vi "requestStop.vi"(8 "error in (no error)":errorcluster, 11 "BoolUserEventStopMechanism In":refnum<class "BoolUserEventStopMechanism.lvclass">) -> (0 "error out":errorcluster, 3 "BoolUserEventStopMechanism Out":refnum<class "BoolUserEventStopMechanism.lvclass">)   [LabVIEW 2023, in "TLC_Daemon.lvlib" / "BoolUserEventStopMechanism.lvclass"]
doc: "Triggers a stop request for a target task.\n_____________________________________\nTLC Daemon 1.0.0.2\nCopyright (c) 2026 Andrea Cadei"
uses:
  BoolUserEventStopMechanism.lvclass
  BoolUserEventStopMechanism.lvclass/BoolUserEventStopMechanism.ctl
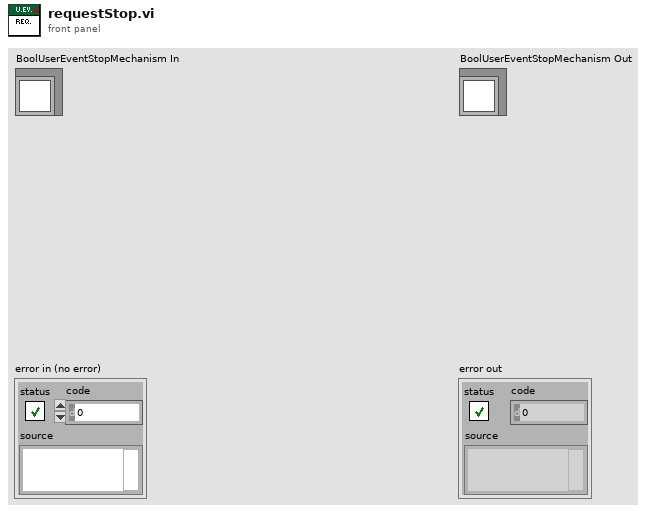
[diagram p1: front panel]
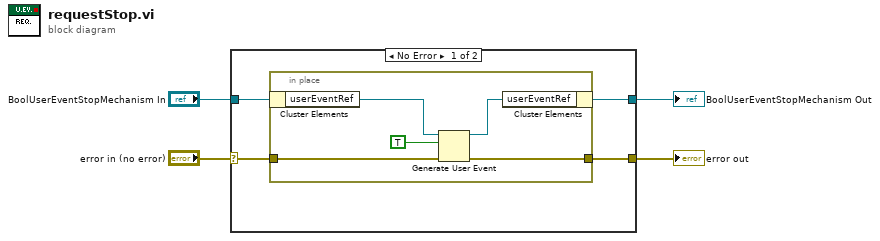
[diagram p0: block diagram]
diagram:
  n1 = case shown="No Error" "error in (no error)" {
    selector: "error in (no error)" -> [w7 w15]
    tunnel: [w6 w15] -> w3
    tunnel: "BoolUserEventStopMechanism In" -> [w8 w14]
    tunnel: [w5 w14] -> w1
    frame No Error {
      n2 = in-place {
        in-place-border: w7 -> [w10]
        in-place-border: [w9] -> w6
        n3 = in-place-cluster #1(w8) -> ("userEventRef"=w13:refnum<user-event>)
        n4 = Generate User Event(user event=w13, event data cluster=TRUE ("notification"), error in=w10) -> (user event out=w12:refnum<user-event>, error out=w9:errorcluster)  [unwired: 1 in]
        n5 = in-place-cluster #1("userEventRef"=w12) -> (w5:refnum<class "BoolUserEventStopMechanism.lvclass">)
      }
    }
    frame Error {
    }
  }
  "error out" <- w3
  "BoolUserEventStopMechanism Out" <- w1
